vi "Grid Generator.vi"(0 "Dimension":i32, 1 "Call Type":enum16{"Reset", "Grid Generator"}(ring), 7 "Upper Limit":dbl=1.0, 9 "Spacing":dbl=0.01, 11 "Lower Limit":dbl) -> (8 "Output":dbl)   [LabVIEW 2011]
panel:
  out "Limits":dbl[][](array[numeric])
  out "Index":i32[](array[numeric])
  out "Subarray":dbl[](array[numeric])
  out "Array":dbl[][](array[numeric])
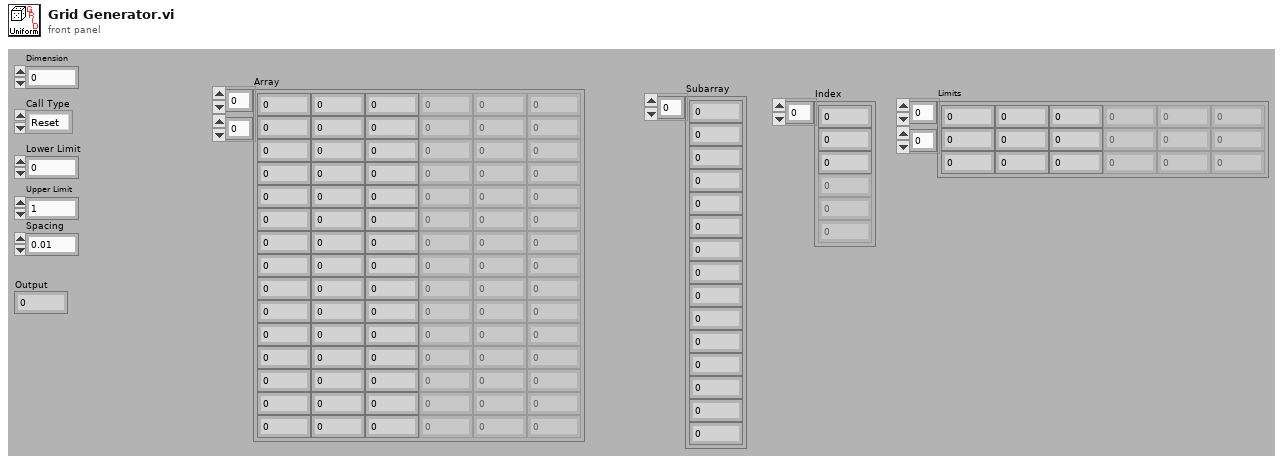
[diagram p1: front panel]
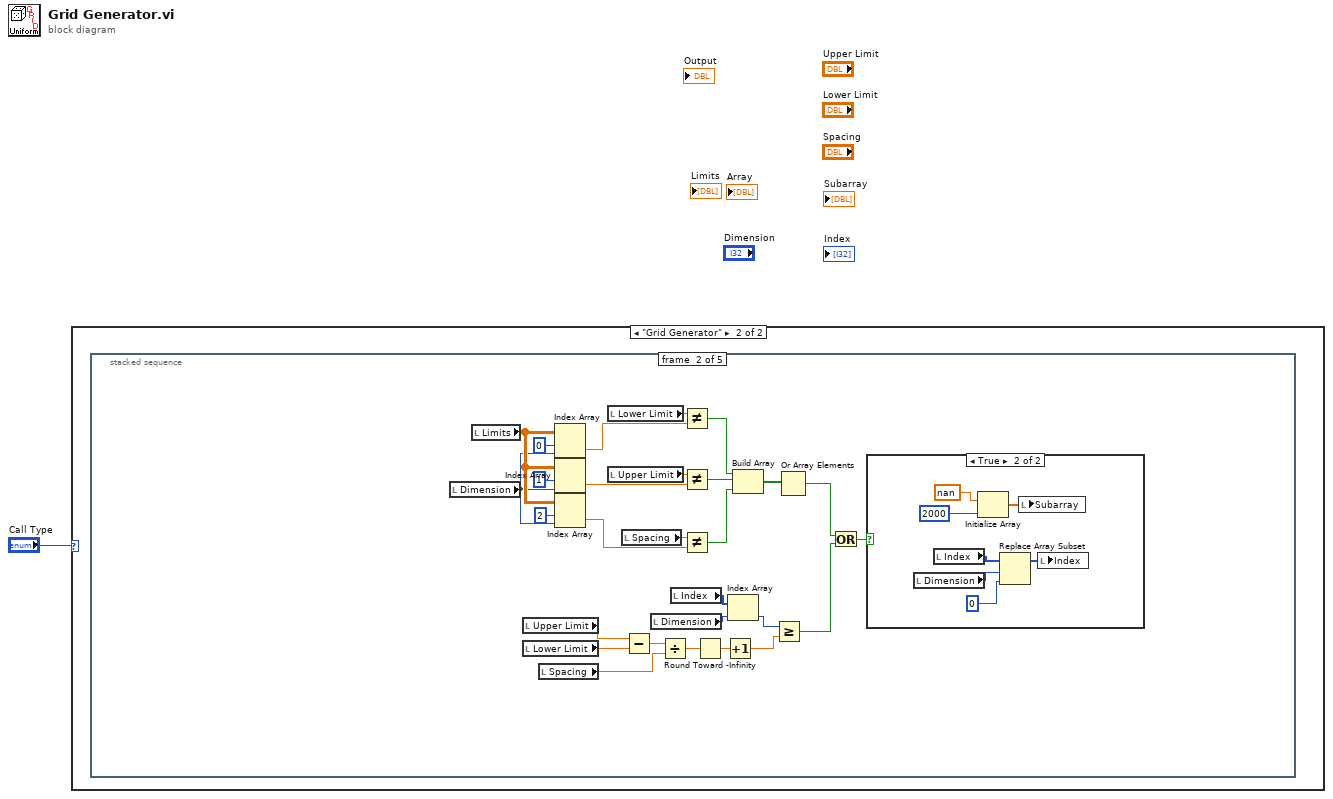
[diagram p0: block diagram]
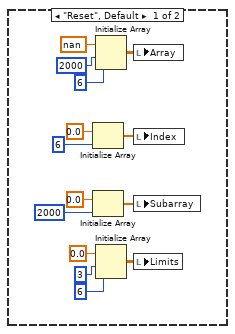
[diagram p2: hidden frame]
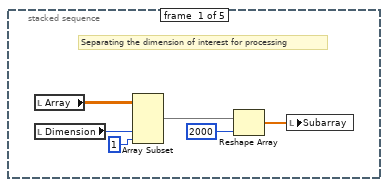
[diagram p3: hidden frame]
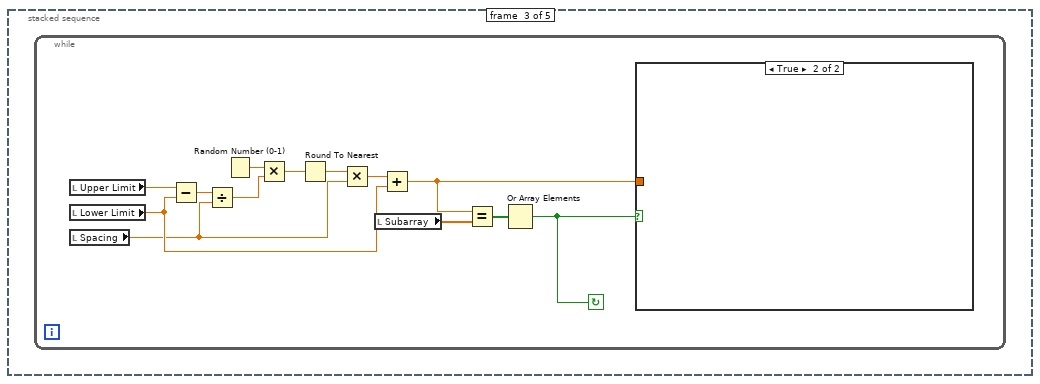
[diagram p5: hidden frame]
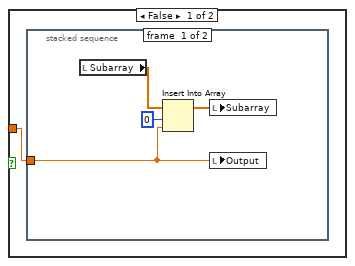
[diagram p6: hidden frame]
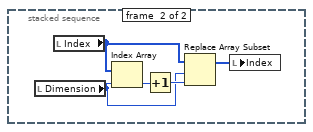
[diagram p7: hidden frame]
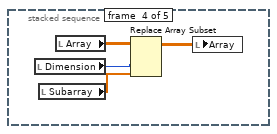
[diagram p8: hidden frame]
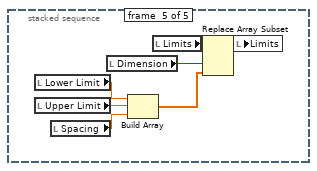
[diagram p9: hidden frame]
diagram:
  n1 = case shown="\"Grid Generator\"" "Call Type" {
    frame "Reset", Default {
      n2 = Initialize Array(0.0 ("element"), 6 ("dimension size")) -> (w9:dbl[])
      n3 = Initialize Array(0.0 ("element"), 2000 ("dimension size")) -> (w8:dbl[])
      n4 = Initialize Array(nan ("element"), 2000 ("dimension size"), 6 ("dimension size")) -> (w15:dbl[][])
      n5 = Initialize Array(0.0 ("element"), 3 ("dimension size"), 6 ("dimension size")) -> (w2:dbl[][])
      n6 = local write "Array"(w15) -> ()
      n7 = local write "Index"(w9) -> ()
      n8 = local write "Subarray"(w8) -> ()
      n9 = local write "Limits"(w2) -> ()
    }
    frame "Grid Generator" {
      n10 = stacked-sequence {
        frame #0 {
          # "Separating the dimension of interest for processing"
          n11 = local read "Array"() -> (w19:dbl[][])
          n12 = local read "Dimension"() -> (w17:i32)
          n13 = Array Subset(array=w19, index (col)=w17, length (col)=1 ("length")) -> (w21:dbl[][])  [unwired: 2 in]
          n14 = Reshape Array(w21, 2000 ("dimension size")) -> (w20:dbl[])
          n15 = local write "Subarray"(w20) -> ()
        }
        frame #1 {
          n16 = local read "Dimension"() -> (w23:i32)
          n17 = local read "Limits"() -> (w29:dbl[][])
          n18 = local read "Upper Limit"() -> (w39:dbl)
          n19 = local read "Lower Limit"() -> (w38:dbl)
          n20 = local read "Spacing"() -> (w37:dbl)
          n21 = Index Array(array=w29, index (row)=0 ("disabled index (row)"), index (col)=w23) -> (element=w28:dbl)
          n22 = Index Array(array=w29, index (row)=1 ("disabled index (row)"), index (col)=w23) -> (element=w27:dbl)
          n23 = Index Array(array=w29, index (row)=2 ("disabled index (row)"), index (col)=w23) -> (element=w26:dbl)
          n24 = local read "Lower Limit"() -> (w45:dbl)
          n25 = local read "Upper Limit"() -> (w44:dbl)
          n26 = local read "Spacing"() -> (w43:dbl)
          n27 = Subtract(x=w39, y=w38) -> (x-y=w40:dbl)
          n28 = local read "Dimension"() -> (w35:i32)
          n29 = Divide(x=w40, y=w37) -> (x/y=w36:dbl)
          n30 = local read "Index"() -> (w34:i32[])
          n31 = Not Equal?(x=w45, y=w28) -> (x != y?=w46:bool)
          n32 = Not Equal?(x=w44, y=w27) -> (x != y?=w47:bool)
          n33 = Not Equal?(x=w43, y=w26) -> (x != y?=w48:bool)
          n34 = Round Toward -Infinity(1:w36) -> (0:w30:dbl)
          n35 = Increment(x=w30) -> (x+1=w31:dbl)
          n36 = Index Array(array=w34, index=w35) -> (element=w33:i32)
          n37 = Build Array(w46, w47, w48) -> (w49:bool[])
          n38 = Greater Or Equal?(x=w33, y=w31) -> (x >= y?=w32:bool)
          n39 = Or Array Elements(Boolean array=w49) -> (logical OR=w42:bool)
          n40 = Or(x=w42, y=w32) -> (x .or. y?=w41:bool)
          n41 = case shown="True" w41 {
            frame False {
            }
            frame True {
              n42 = local read "Dimension"() -> (w54:i32)
              n43 = local read "Index"() -> (w56:i32[])
              n44 = Initialize Array(nan ("element"), 2000 ("dimension size")) -> (w50:dbl[])
              n45 = Replace Array Subset(array=w56, new element=0 ("new element/subarray"), index=w54) -> (w53:i32[])
              n46 = local write "Subarray"(w50) -> ()
              n47 = local write "Index"(w53) -> ()
            }
          }
        }
        frame #2 {
          n48 = while {
            stop <- w69 continue-if-true
            n49 = local read "Upper Limit"() -> (w62:dbl)
            n50 = local read "Lower Limit"() -> (w61:dbl)
            n51 = local read "Spacing"() -> (w60:dbl)
            n52 = Subtract(x=w62, y=w61) -> (x-y=w67:dbl)
            n53 = Divide(x=w67, y=w60) -> (x/y=w63:dbl)
            n54 = Random Number (0-1)() -> (number: 0 to 1=w68:dbl)
            n55 = Multiply(x=w68, y=w63) -> (x*y=w65:dbl)
            n56 = Round To Nearest(number=w65) -> (nearest integer value=w64:dbl)
            n57 = Multiply(x=w64, y=w60) -> (x*y=w66:dbl)
            n58 = local read "Subarray"() -> (w58:dbl[])
            n59 = Add(x=w66, y=w61) -> (x+y=w59:dbl)
            n60 = Equal?(x=w59, y=w58) -> (x = y?=w57:bool[])
            n61 = Or Array Elements(Boolean array=w57) -> (logical OR=w69:bool)
            n62 = case shown="True" w69 {
              tunnel: w59 -> [w70 _]
              frame False {
                n63 = stacked-sequence {
                  tunnel: w70 -> [w72 _]
                  frame #0 {
                    n64 = local read "Subarray"() -> (w74:dbl[])
                    n65 = Insert Into Array(array=w74, index=0, new element=w72) -> (w73:dbl[])
                    n66 = local write "Subarray"(w73) -> ()
                    n67 = local write "Output"(w72) -> ()
                  }
                  frame #1 {
                    n68 = local read "Dimension"() -> (w77:i32)
                    n69 = local read "Index"() -> (w76:i32[])
                    n70 = Index Array(array=w76, index=w77) -> (element=w79:i32)
                    n71 = Increment(x=w79) -> (x+1=w78:i32)
                    n72 = Replace Array Subset(array=w76, new element=w78, index=w77) -> (w75:i32[])
                    n73 = local write "Index"(w75) -> ()
                  }
                }
              }
              frame True {
              }
            }
          }
        }
        frame #3 {
          n74 = local read "Dimension"() -> (w80:i32)
          n75 = local read "Subarray"() -> (w81:dbl[])
          n76 = local read "Array"() -> (w83:dbl[][])
          n77 = Replace Array Subset(array=w83, new element=w81, index (col)=w80) -> (w82:dbl[][])  [unwired: 1 in]
          n78 = local write "Array"(w82) -> ()
        }
        frame #4 {
          n79 = local read "Lower Limit"() -> (w88:dbl)
          n80 = local read "Upper Limit"() -> (w87:dbl)
          n81 = local read "Spacing"() -> (w86:dbl)
          n82 = local read "Dimension"() -> (w89:i32)
          n83 = Build Array(w88, w87, w86) -> (w85:dbl[])
          n84 = local read "Limits"() -> (w84:dbl[][])
          n85 = Replace Array Subset(array=w84, new element=w85, index (col)=w89) -> (w90:dbl[][])  [unwired: 1 in]
          n86 = local write "Limits"(w90) -> ()
        }
      }
    }
  }
